vi "MM6Archiver.new event data.vi"(0 "i ref":refnum<vi>, 1 "eventData":string, 2 "descriptor":string, 3 "ms timeout (10000)":i32=10000, 5 "error in (no error)":errorcluster) -> (14 "i ref out":refnum<vi>, 17 "timed out":bool, 19 "error out":errorcluster)   [LabVIEW 2014, in "MM6Archiver.lvlib"]
doc: "The method is executed, when new event data is received. The data will be written to file."
uses:
  MM6Archiver.lvlib
  CSCore/CSSystem/CoreDefs/CoreDefs.rawDataType.ctl
  CSCore/CSSystem/CoreDefs/CoreDefs.error_type.ctl
  CSCore/CSSystem/CoreDefs/CoreDefs.error_severity.ctl
  CSData/DiscArchiver/DiscArchiver.lvlib
  CSData/DataLib/DataLib.lvlib
  CSCore/CSSystem/CoreLib/CoreLib.lvlib
  CSlibraries-extern/DimLVEvent/LVDimInterface/LVDimInterface.lvlib
  CSlibraries/UtilityLib/UtilityLib.lvlib
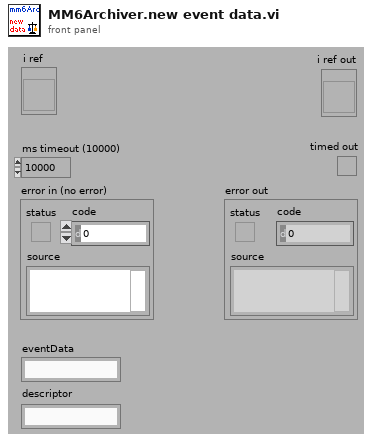
[diagram p1: front panel]
types:
  T1 = typedef "CoreDefs.rawDataType.ctl" = i8[]
  T2 = typedef "CoreDefs.error_severity.ctl" = enum16{"undefined", "information", "warning", "error", "fatal"}
  T3 = typedef "CoreDefs.error_type.ctl" = enum16{"no error", "can't load process", "can't unload process", "process does not exist", "can't install process", "can't remove process", "unknown function", "time out", "can't execute function", "duplicate queue name", "super not found", "caller queue invalid", "can't ping process", "unknown error", "VISA Error", "VISA timeout", "GPIB timeout", "GPIB error", "communication error", "data type mismatch", "can't read data from OPC server", "can't write data to OPC server", "OET error", "function not implemented", "process already exists", "invalid Shared Variable name", "error writing Shared Variable", "error reading Shared Variable", "invalid client name", "corrupt database", "unknown class", "call not authorized", "parameter out of range", "OET timeout: can't get data to modify", "invalid queue name", "requested operation incompatible with current state", "event undefined", "event disabled", "state undefined", "caller is not a friend", "EventBuilder: bad eventID", "EventBuilder: no DAQ devices", "a thread must not stop itself", "UNUSED ELEMENT4", "DiscArchiver: eventData incomplete", "DiscArchiver: eventData does not belong to run", "DiscArchiver: can't open file", "DiscArchiver: can't write to file", "DiscArchiver: available disc space low", "can't acquire semaphore", "error reading data from database", "notifier object is not existing", "can't register process", "can't unregister process", "illegal event type", "object disabled", "object already exists", "can't change state", "Instrument not found", "no connection to remote node", "invalid reference", "N/A", "UNUSED ELEMENT 1", "element not found", "illegal TCP/IP connection detected", "object does not exist", "invalid access ID", "unknown CS system", "invalid privilige", "unsupported data type", "unsupported server type", "IO server already exists", "Shared Variable already exists"}
  T4 = typedef "DiscArchiver.lvlib/DiscArchiver.i attribute.ctl" = cluster{"file prefix":string, "actual file":string, "nOfEvents":i32, "file":refnum<file>, "eventBuilder":string, "disc size alarm":bool, "dataDescription":string, "dataDescriptionURL":string, "eventDataURL":string, "headerID":dbl, "completeData":bool, "nOfEventsID":i32, "dataFileID":i32}
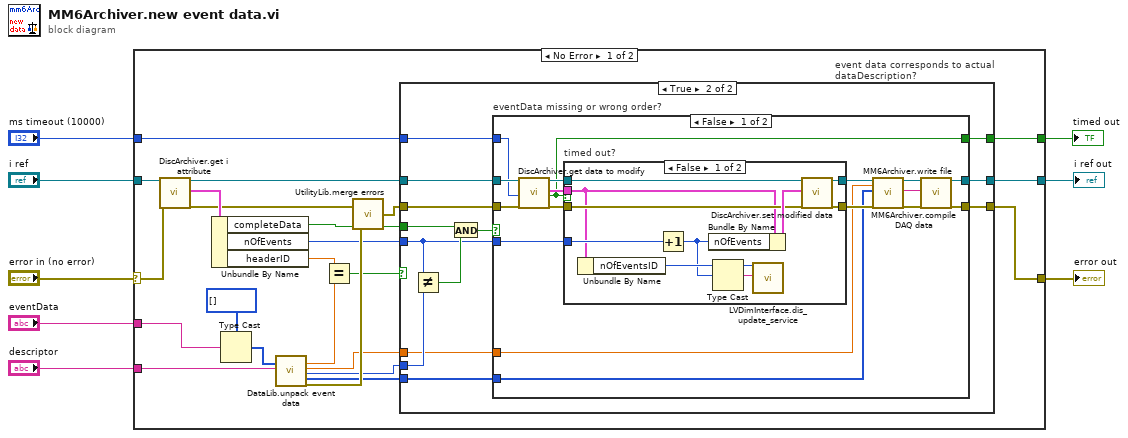
[diagram p0: block diagram]
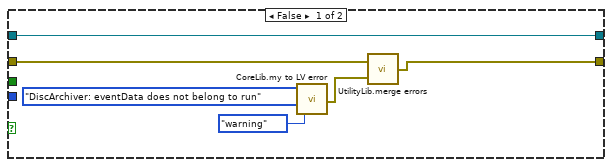
[diagram p2: hidden frame]
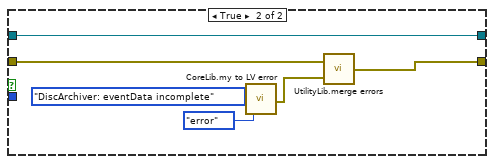
[diagram p4: hidden frame]
diagram:
  n1 = case shown="No Error" "error in (no error)" {
    selector: "error in (no error)" -> [w28 w86]
    tunnel: [w25 w86] -> w8
    tunnel: "eventData" -> [w11 _]
    tunnel: [w24 w87] -> w6
    tunnel: "i ref" -> [w29 w87]
    tunnel: "ms timeout (10000)" -> [w26 _]
    tunnel: "descriptor" -> [w19 _]
    tunnel: [w23 _] -> w2
    frame No Error {
      n2 = call "DiscArchiver.get i attribute.vi"("i ref in"=w29, "error in (no error)"=w28) -> ("i ref out"=w27:refnum<vi>, "i attribute"=w30:T4, "error out"=w17:errorcluster)  [unwired: 15 in]
      n3 = Unbundle By Name(w30) -> ("completeData"=w12:bool, "nOfEvents"=w14:i32, "headerID"=w31:dbl)
      n4 = Type Cast(type=T1 [] ("Array"), x=w11) -> (*(type *) &x=w22:T1)
      n5 = call "DataLib.unpack event data.vi"("serviceData"=w22, "descriptor"=w19) -> ("headerID"=w20:dbl, "timestamp"=w9:dbl, "eventID"=w13:i32, "subEventData"=w10:T1, "error out"=w16:errorcluster)  [unwired: 13 in]
      n6 = Equal?(x=w31, y=w20) -> (x = y?=w15:bool)
      n7 = call "UtilityLib.merge errors.vi"("error2 (no error)"=w16, "error1 (no error)"=w17) -> ("error out"=w18:errorcluster)
      n8 = case "event data corresponds to actual dataDescription?" shown="True" w15 {
        tunnel: w27 -> [w37 w50]
        tunnel: w18 -> [w34 w49]
        tunnel: w26 -> [_ w48]
        tunnel: [w35 w47] -> w25
        tunnel: [w37 w46] -> w24
        tunnel: [_ w45] -> w23
        tunnel: w14 -> [_ w40]
        tunnel: w13 -> [_ w44]
        tunnel: w12 -> [_ w43]
        tunnel: w10 -> [_ w39]
        tunnel: w9 -> [_ w38]
        frame False {
          n9 = call "CoreLib.my to LV error.vi"("ErrorTypes"=CoreDefs.error_type."DiscArchiver: eventData does not belong to run", "severityLevel"=CoreDefs.error_severity."warning") -> ("myErrorCluster"=w33:errorcluster)  [unwired: 16 in, 1 out]
          n10 = call "UtilityLib.merge errors.vi"("error2 (no error)"=w33, "error1 (no error)"=w34) -> ("error out"=w35:errorcluster)
        }
        frame True {
          n11 = Not Equal?(x=w40, y=w44) -> (x != y?=w42:bool)
          n12 = And(x=w43, y=w42) -> (x .and. y?=w41:bool)
          n13 = case "eventData missing or wrong order?" shown="False" w41 {
            tunnel: w50 -> [w67 w85]
            tunnel: w49 -> [w66 w83]
            tunnel: w48 -> [w62 _]
            tunnel: [w61 w84] -> w47
            tunnel: [w60 w85] -> w46
            tunnel: [w58 _] -> w45
            tunnel: w40 -> [w59 _]
            tunnel: w39 -> [w52 _]
            tunnel: w38 -> [w51 _]
            frame False {
              n14 = call "DiscArchiver.get data to modify.vi"("i ref in"=w67, "ms timeout (10000)"=w62, "error in (no error)"=w66) -> ("i ref out"=w65:refnum<vi>, "i attribute"=w64:T4, "timed out"=w58:bool, "error out"=w63:errorcluster)  [unwired: 13 in]
              n15 = case "timed out?" shown="False" w58 {
                tunnel: w65 -> [w77 w78]
                tunnel: w64 -> [w71 _]
                tunnel: w63 -> [w75 w79]
                tunnel: [w72 w79] -> w56
                tunnel: [w74 w78] -> w57
                tunnel: w59 -> [w73 _]
                frame False {
                  n16 = Unbundle By Name(w71) -> ("nOfEventsID"=w70:i32)
                  n17 = Increment(x=w73) -> (x+1=w68:i32)
                  n18 = Bundle By Name(cluster=w71, "nOfEvents"=w68) -> (w76:T4)
                  n19 = Type Cast(x=w68) -> (*(type *) &x=w69:string)  [unwired: 1 in]
                  n20 = call "LVDimInterface.dis_update_service.vi"("my_serviceID"=w70, "data"=w69) -> ()  [unwired: 15 in, 3 out]
                  n21 = call "DiscArchiver.set modified data.vi"("i ref in"=w77, "i attribute"=w76, "error in (no error)"=w75) -> ("i ref out"=w74:refnum<vi>, "error out"=w72:errorcluster)  [unwired: 15 in]
                }
                frame True {
                }
              }
              n22 = call "MM6Archiver.compile DAQ data.vi"("i ref in"=w57, "timeStamp"=w51, "eventData"=w52, "error in (no error)"=w56) -> ("i ref out"=w54:refnum<vi>, "trapData"=w55:string, "error out"=w53:errorcluster)  [unwired: 13 in]
              n23 = call "MM6Archiver.write file.vi"("i ref in"=w54, "eventData"=w55, "error in (no error)"=w53) -> ("i ref out"=w60:refnum<vi>, "error out"=w61:errorcluster)  [unwired: 15 in]
            }
            frame True {
              n24 = call "CoreLib.my to LV error.vi"("ErrorTypes"=CoreDefs.error_type."DiscArchiver: eventData incomplete", "severityLevel"=CoreDefs.error_severity."error") -> ("myErrorCluster"=w82:errorcluster)  [unwired: 16 in, 1 out]
              n25 = call "UtilityLib.merge errors.vi"("error2 (no error)"=w82, "error1 (no error)"=w83) -> ("error out"=w84:errorcluster)
            }
          }
        }
      }
    }
    frame Error {
    }
  }
  "error out" <- w8
  "i ref out" <- w6
  "timed out" <- w2
